vi "DAQ comm.vi"(7 "DAQ cluster in":T1 {"temp"."utility"."therm volt" format="%_6g"; "temp"."utility"."heat volt in" format="%_6g"; "temp"."utility"."heat volt out" format="%_6g"; "temp"."utility"."power out" format="%_6g"; "temp"."utility"."H Vmax" format="%_6g"; "temp"."T exec"."man power" format="%_6g"; "temp"."T exec"."exec setpoint" format="%_6g"; "temp"."T params"."Settle Time" step=1.0; "temp"."T params"."Settle Bandwidth" step=0.01; "temp"."T params"."Derivative Tme" step=0.01; "temp"."T params"."Integral Time" step=1.0; "temp"."T params"."Control Bandwidth" step=0.1; "temp"."T params"."Setpoint" step=0.1; "temp"."T status"."Setpoint" format="%_6g"; "temp"."T status"."Power" format="%_6g"; "temp"."T status"."Temp" format="%_6g"}) -> (8 "DAQ cluster out":T1 {"temp"."utility"."therm volt" format="%_6g"; "temp"."utility"."heat volt in" format="%_6g"; "temp"."utility"."heat volt out" format="%_6g"; "temp"."utility"."power out" format="%_6g"; "temp"."utility"."H Vmax" format="%_6g"; "temp"."T exec"."man power" format="%_6g"; "temp"."T exec"."exec setpoint" format="%_6g"; "temp"."T params"."Settle Time" step=1.0; "temp"."T params"."Settle Bandwidth" step=0.01; "temp"."T params"."Derivative Tme" step=0.01; "temp"."T params"."Integral Time" step=1.0; "temp"."T params"."Control Bandwidth" step=0.1; "temp"."T params"."Setpoint" step=0.1; "temp"."T status"."Setpoint" format="%_6g"; "temp"."T status"."Power" format="%_6g"; "temp"."T status"."Temp" format="%_6g"})   [LabVIEW 2019]
doc: "This subVI is one of the states of the DAQ state machine in the bug experiment.\n\nThis state monitors and maintains the global variables used in the bug experiment. It also clear the measurement on changing from settle to measurment mode or back the other way.\n\nPaul K Dixon\nP3600\nCSUSB Physics"
uses:
  typedefs/DAQ state cluster.ctl
  typedefs/DAQ state enum.ctl
  typedefs/temp cont cluster.ctl
  typedefs/temp exec cluster.ctl
  typedefs/temp mode enum.ctl
  typedefs/temp indicator.ctl
  typedefs/temp control status.ctl
  typedefs/PID control parameters.ctl
  typedefs/temp cont utility.ctl
  typedefs/measurement.ctl
  typedefs/wvfm acq params.ctl
  globals/Bug globals.vi
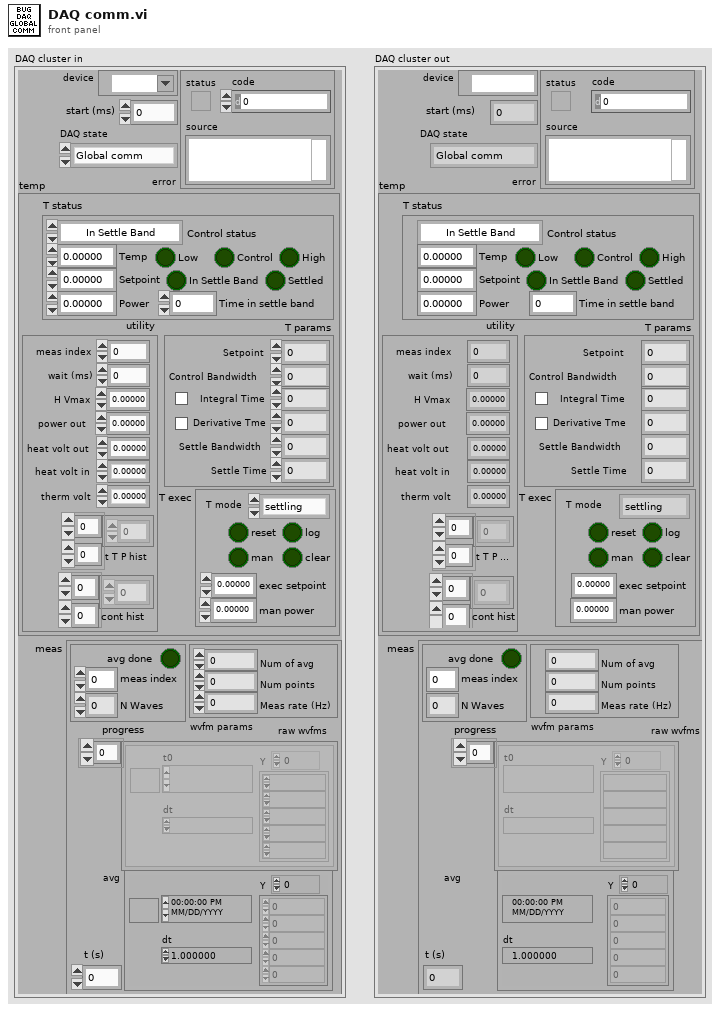
[diagram p1: front panel]
types:
  T1 = typedef "DAQ state cluster.ctl" = cluster{"DAQ state":T2, "temp":T3, "meas":T10, "device":tag, "error":errorcluster, "start (ms)":i32}
  T2 = typedef "DAQ state enum.ctl" = enum16{"Global comm", "Meas T & P", "PID power calc", "Man Power set", "Output Power", "Wait", "Meas wvfm", "Avg wvfm", "Exit"}
  T3 = typedef "temp cont cluster.ctl" = cluster{"T exec":T4, "T status":T6, "T params":T8, "utility":T9}
  T4 = typedef "temp exec cluster.ctl" = cluster{"T mode":T5, "exec setpoint":dbl, "reset":bool, "man power":dbl, "man":bool, "log":bool, "clear":bool}
  T5 = typedef "temp mode enum.ctl" = enum16{"settling", "measuring", "holding", "Exit"}
  T6 = typedef "temp indicator.ctl" = cluster{"Control status":T7, "Temp":dbl, "Power":dbl, "Time in settle band":dbl, "Settled":bool, "Low":bool, "High":bool, "Setpoint":dbl, "Control":bool, "In Settle Band":bool}
  T7 = typedef "temp control status.ctl" = enum16{"In Settle Band", "In Control Band", "Below Control Band", "Above Control Band"}
  T8 = typedef "PID control parameters.ctl" = cluster{"Setpoint":dbl, "Control Bandwidth":dbl, "Integral Time":dbl, "Int\nON":bool, "Derivative Tme":dbl, "Der\nON":bool, "Settle Bandwidth":dbl, "Settle Time":dbl}
  T9 = typedef "temp cont utility.ctl" = cluster{"meas index":i32, "wait (ms)":i32, "H Vmax":dbl, "power out":dbl, "heat volt out":dbl, "heat volt in":dbl, "therm volt":dbl, "t T P hist":dbl[][], "cont hist":dbl[][]}
  T10 = typedef "measurement.ctl" = cluster{"wvfm params":T11, "avg":waveform(dbl), "raw wvfms":waveform(dbl)[], "progress":cluster{"avg done":bool, "meas index":i32, "N waves":i32}, "t (s)":dbl}
  T11 = typedef "wvfm acq params.ctl" = cluster{"Num of avg":i32, "Num points":i32, "Meas rate (Hz)":dbl}
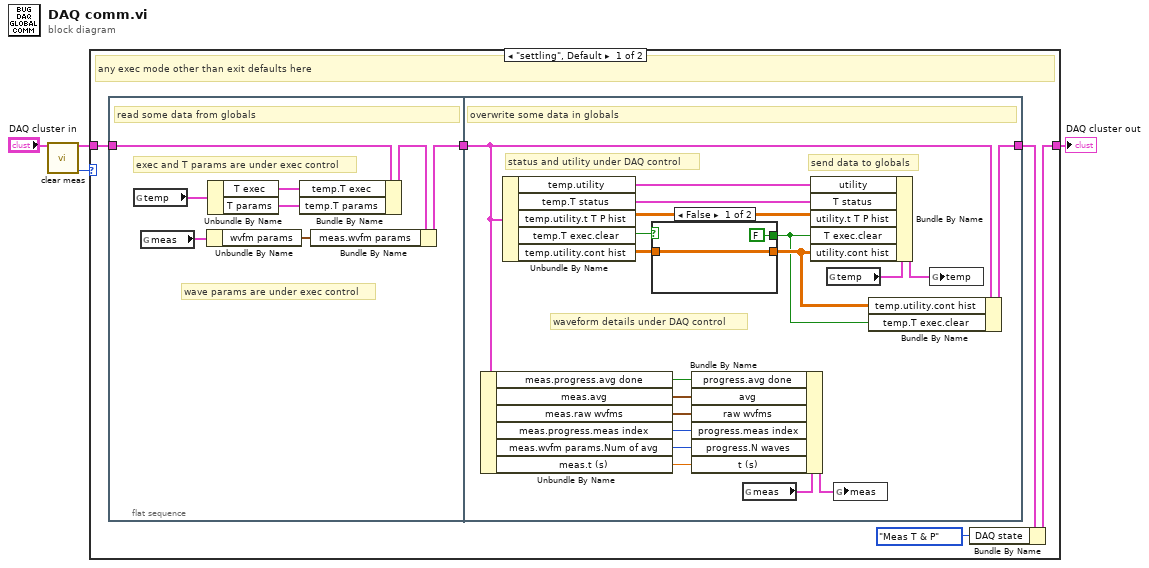
[diagram p0: block diagram]
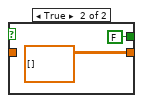
[diagram p2: hidden frame]
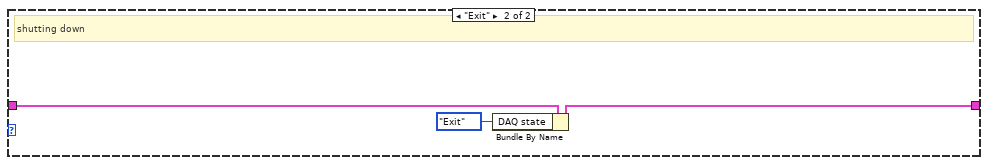
[diagram p3: hidden frame]
diagram:
  n1 = call "clear meas.vi"("DAQ cluster in"="DAQ cluster in") -> ("DAQ cluster out"=w2:T1, "T mode out"=w1:T5)  [unwired: 13 in]
  n2 = case shown="\"settling\", Default" w1 {
    tunnel: w2 -> [w9 w43]
    tunnel: [w8 w42] -> w4
    frame "settling", Default {
      # "any exec mode other than exit defaults here"
      n3 = flat-sequence {
        tunnel: w9 -> [w17]
        tunnel: [w13] -> w6
        tunnel: [w30] -> w7
        tunnel: w6 -> [w26]
        frame #0 {
          # "wave params are under exec control"
          # "exec and T params are under exec control"
          # "read some data from globals"
          n4 = global read "Bug globals.vi" "temp"() -> (w12:T3)
          n5 = global read "Bug globals.vi" "meas"() -> (w11:T10)
          n6 = Unbundle By Name(w11) -> ("wvfm params"=w10:T11)
          n7 = Unbundle By Name(w12) -> ("T exec"=w16:T4, "T params"=w15:T8)
          n8 = Bundle By Name(cluster=w17, "temp.T exec"=w16, "temp.T params"=w15) -> (w14:T1)
          n9 = Bundle By Name(cluster=w14, "meas.wvfm params"=w10) -> (w13:T1)
        }
        frame #1 {
          # "waveform details under DAQ control"
          # "status and utility under DAQ control"
          # "send data to globals"
          # "overwrite some data in globals"
          n10 = Unbundle By Name(w26) -> ("meas.progress.avg done"=w19:bool, "meas.avg"=w23:waveform(dbl), "meas.raw wvfms"=w22:waveform(dbl)[], "meas.progress.meas index"=w21:i32, "meas.wvfm params.Num of avg"=w20:i32, "meas.t (s)"=w18:dbl)
          n11 = Unbundle By Name(w26) -> ("temp.utility"=w27:T9, "temp.T status"=w34:T6, "temp.utility.t T P hist"=w33:dbl[][], "temp.T exec.clear"=w32:bool, "temp.utility.cont hist"=w31:dbl[][])
          n12 = case shown="False" w32 {
            tunnel: [FALSE FALSE] -> w28
            tunnel: [w38 dbl[][] [] ("f")] -> w29
            tunnel: w31 -> [w38 _]
            frame False {
            }
            frame True {
            }
          }
          n13 = global read "Bug globals.vi" "meas"() -> (w25:T10)
          n14 = Bundle By Name(cluster=w25, "progress.avg done"=w19, "avg"=w23, "raw wvfms"=w22, "progress.meas index"=w21, "progress.N waves"=w20, "t (s)"=w18) -> (w24:T10)
          n15 = global read "Bug globals.vi" "temp"() -> (w36:T3)
          n16 = Bundle By Name(cluster=w36, "utility"=w27, "T status"=w34, "utility.t T P hist"=w33, "T exec.clear"=w28, "utility.cont hist"=w29) -> (w35:T3)
          n17 = global write "Bug globals.vi" "meas"(w24) -> ()
          n18 = Bundle By Name(cluster=w26, "temp.utility.cont hist"=w29, "temp.T exec.clear"=w28) -> (w30:T1)
          n19 = global write "Bug globals.vi" "temp"(w35) -> ()
        }
      }
      n20 = Bundle By Name(cluster=w7, "DAQ state"=DAQ_state_enum."Meas T & P") -> (w8:T1)
    }
    frame "Exit" {
      # "shutting down"
      n21 = Bundle By Name(cluster=w43, "DAQ state"=DAQ_state_enum."Exit") -> (w42:T1)
    }
  }
  "DAQ cluster out" <- w4
